vi "addADCOffsetSensitivityFrame.vi"(8 "error in (no error)":errorcluster, 10 "ModbusBuffer in":refnum<class "ModbusBuffer.lvclass">, 11 "ILC in":refnum<class "ILC.lvclass">) -> (0 "error out":errorcluster, 2 "ModbusBuffer out":refnum<class "ModbusBuffer.lvclass">, 3 "ILC out":refnum<class "ILC.lvclass">)   [LabVIEW 2016, in "RTILC.lvlib" / "ILC.lvclass"]
uses:
  ILC.lvclass
  Common_RT_Modbus/ModbusBuffer/ModbusBuffer.lvclass
  ILC.lvclass/ILC.ctl
  Common_RT_Modbus/DataTypes/ExceptionCodes.ctl
  Common_RT_Modbus/ModbusBuffer/ModbusBuffer.lvclass/ModbusBuffer.ctl
  Common_RT_Modbus/ModbusBuffer/writeByteInstruction.vi
  Common_RT_Modbus/ModbusBuffer/calculateCRC.vi
  Common_RT_Modbus/RTModbus.lvlib
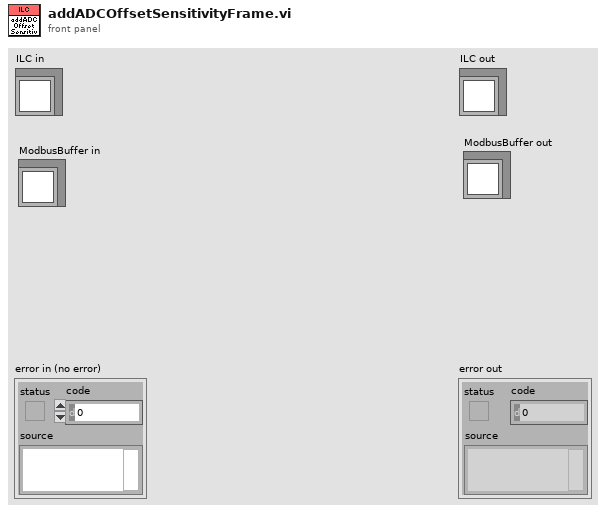
[diagram p1: front panel]
types:
  T1 = typedef "RTModbus.lvlib/ExceptionCodes.ctl" = u16
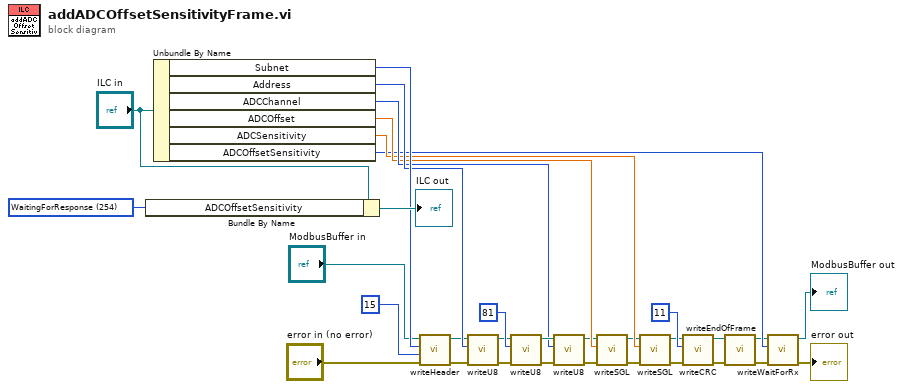
[diagram p0: block diagram]
diagram:
  w31 = T1 254 items=["OK"=0, "IllegalFunction"=1, "IllegalDataAddress"=2, "IllegalDataValue"=3, "SlaveDeviceFailure"=4, "Acknowledge"=5, "SlaveDeviceBusy"=6, "NegativeAcknowledge"=7, "MemoryParityError"=8, "GatewayPathUnavailable"=9, "GatewayTargetDeviceFailedToRespond"=10, "WaitingForResponse"=254, "CRCError"=255] ("ILCData.Responses.ADCOffsetSensitivity")
  n1 = Bundle By Name(cluster="ILC in", "ADCOffsetSensitivity"=w31) -> (→"ILC out":refnum<class "ILC.lvclass">)
  n2 = Unbundle By Name("ILC in") -> ("Subnet"=w27:u8, "Address"=w25:u8, "ADCChannel"=w23:u8, "ADCOffset"=w22:sgl, "ADCSensitivity"=w21:sgl, "ADCOffsetSensitivity"=w19:u32)
  n3 = call "writeHeader.vi"("error in (no error)"="error in (no error)", "Length"=u16 15, "Subnet"=w27, "ModbusBuffer in"="ModbusBuffer in") -> ("error out"=w8:errorcluster, "ModbusBuffer out"=w17:refnum<class "ModbusBuffer.lvclass">)  [unwired: 6 in]
  n4 = call "writeU8.vi"("error in (no error)"=w8, "Input"=w25, "ModbusBuffer in"=w17) -> ("error out"=w7:errorcluster, "ModbusBuffer out"=w16:refnum<class "ModbusBuffer.lvclass">)  [unwired: 7 in]
  n5 = call "writeU8.vi"("error in (no error)"=w7, "Input"=u8 81 ("Byte"), "ModbusBuffer in"=w16) -> ("error out"=w29:errorcluster, "ModbusBuffer out"=w28:refnum<class "ModbusBuffer.lvclass">)  [unwired: 7 in]
  n6 = call "writeU8.vi"("error in (no error)"=w29, "Input"=w23, "ModbusBuffer in"=w28) -> ("error out"=w6:errorcluster, "ModbusBuffer out"=w15:refnum<class "ModbusBuffer.lvclass">)  [unwired: 7 in]
  n7 = call "writeSGL.vi"("error in (no error)"=w6, "Input"=w22, "ModbusBuffer in"=w15) -> ("error out"=w5:errorcluster, "ModbusBuffer out"=w14:refnum<class "ModbusBuffer.lvclass">)  [unwired: 7 in]
  n8 = call "writeSGL.vi"("error in (no error)"=w5, "Input"=w21, "ModbusBuffer in"=w14) -> ("error out"=w4:errorcluster, "ModbusBuffer out"=w13:refnum<class "ModbusBuffer.lvclass">)  [unwired: 7 in]
  n9 = call "writeCRC.vi"("error in (no error)"=w4, "Length"=11, "ModbusBuffer in"=w13) -> ("error out"=w3:errorcluster, "ModbusBuffer out"=w12:refnum<class "ModbusBuffer.lvclass">)  [unwired: 7 in]
  n10 = call "writeEndOfFrame.vi"("error in (no error)"=w3, "ModbusBuffer in"=w12) -> ("error out"=w2:errorcluster, "ModbusBuffer out"=w11:refnum<class "ModbusBuffer.lvclass">)  [unwired: 8 in]
  n11 = call "writeWaitForRx.vi"("error in (no error)"=w2, "Timeout(us)"=w19, "ModbusBuffer in"=w11) -> ("error out"=→"error out":errorcluster, "ModbusBuffer out"=→"ModbusBuffer out":refnum<class "ModbusBuffer.lvclass">)  [unwired: 7 in]
